vi "validate line configuration.vi"(7 "module":refnum<class "PID Module configuration.lvclass">, 10 "old loop in (optional)":T1={"Loop ID"="", "Tags"={"Setpoint"="", "Process Variable"="", "Output"=""}, "Gains"={"P"=1.0, "I"=0.01, "D"=0.0}, "Range"={"High"=100.0, "Low"=-100.0}}, 11 "new loop in":T1={"Loop ID"="", "Tags"={"Setpoint"="", "Process Variable"="", "Output"=""}, "Gains"={"P"=1.0, "I"=0.01, "D"=0.0}, "Range"={"High"=100.0, "Low"=-100.0}}) -> (1 "valid?":bool, 2 "errors":string, 3 "new loop out":T1={"Loop ID"="", "Tags"={"Setpoint"="", "Process Variable"="", "Output"=""}, "Gains"={"P"=1.0, "I"=0.01, "D"=0.0}, "Range"={"High"=100.0, "Low"=-100.0}})   [LabVIEW 2013, in "PID Module editor node.lvclass"]
uses:
  PID Module editor node.lvclass
  PID array element.ctl
  module/configuration/PID Module configuration.lvclass
  module/configuration/PID Loop/PID Loop.lvclass
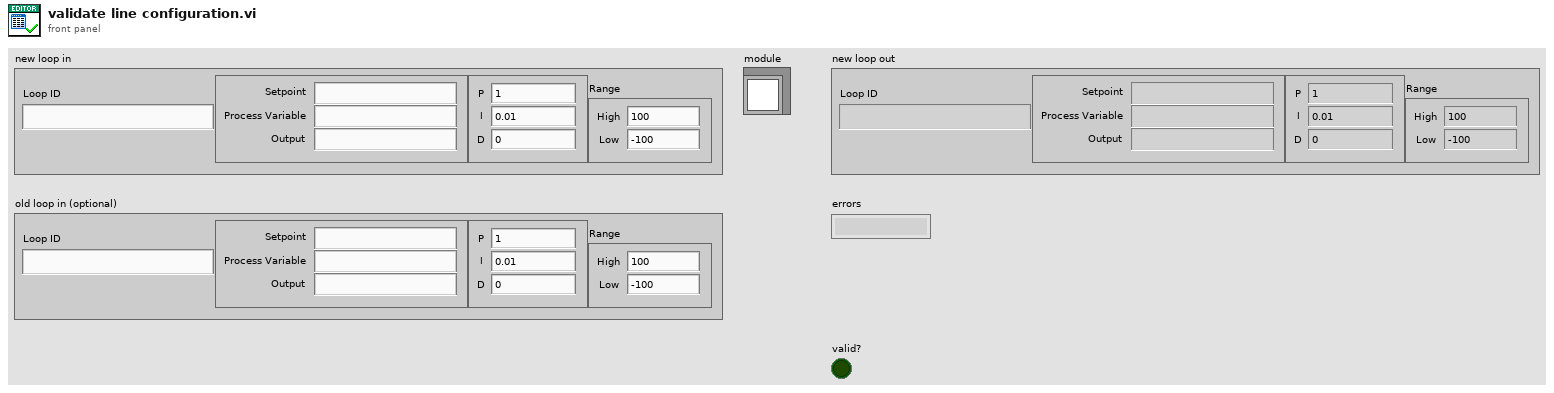
[diagram p1: front panel]
types:
  T1 = typedef "PID Module configuration.lvclass/PID array element.ctl" = cluster{"Loop ID":string, "Tags":cluster{"Setpoint":string, "Process Variable":string, "Output":string}, "Gains":cluster{"P":dbl, "I":dbl, "D":dbl}, "Range":cluster{"High":dbl, "Low":dbl}}
  T2 = typedef "PID Loop.lvclass/PID Parameters.ctl" = cluster{"Setpoint Tag":string, "Process Variable Tag":string, "Output Tag":string}
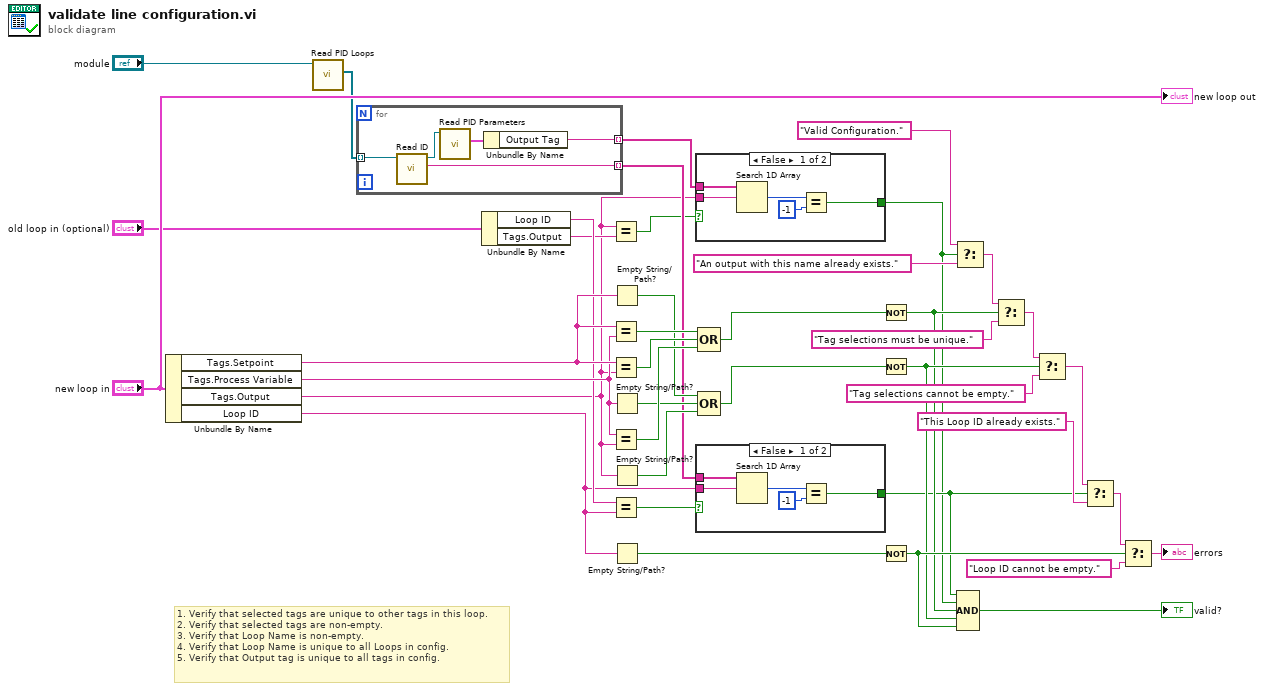
[diagram p0: block diagram]
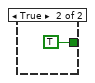
[diagram p2: hidden frame]
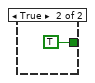
[diagram p3: hidden frame]
diagram:
  # "1. Verify that selected tags are unique to other tags in this loop.\n2. Verify that selected tags are non-empty.\n3. Verify that Loop Name is non-empty.\n4. Verify that Loop Name is unique to all Loops in config.\n5. Verify that Output tag is unique to all tags in config."
  n1 = Unbundle By Name("new loop in") -> ("Tags.Setpoint"=w36:string, "Tags.Process Variable"=w35:string, "Tags.Output"=w4:string, "Loop ID"=w7:string)
  n2 = call-dynamic "Read PID Loops.vi"("Tagbus PID Module configuration in"="module") -> ("PID Loops"=w1:refnum<class "PID Loop.lvclass">[])  [unwired: 8 in, 2 out]
  n3 = for {
    tunnel: w1 -> [w44] mode=indexing
    tunnel: [w43] -> w13 mode=indexing
    tunnel: [w45] -> w11 mode=indexing
    n4 = call-dynamic "Read ID.vi"("PID Loop in"=w44) -> ("ID"=w43:string, "PID Loop out"=w42:refnum<class "PID Loop.lvclass">)  [unwired: 8 in, 1 out]
    n5 = call-dynamic "Read PID Parameters.vi"("PID Loop in"=w42) -> ("PID Parameters"=w41:T2)  [unwired: 8 in, 2 out]
    n6 = Unbundle By Name(w41) -> ("Output Tag"=w45:string)
  }
  n7 = Unbundle By Name("old loop in (optional)") -> ("Loop ID"=w8:string, "Tags.Output"=w5:string)
  n8 = Equal?(x=w4, y=w5) -> (x = y?=w3:bool)
  n9 = Equal?(x=w36, y=w35) -> (x = y?=w39:bool)
  n10 = Equal?(x=w36, y=w4) -> (x = y?=w38:bool)
  n11 = Equal?(x=w35, y=w4) -> (x = y?=w37:bool)
  n12 = Equal?(x=w8, y=w7) -> (x = y?=w6:bool)
  n13 = Empty String/Path?(string/path=w36) -> (empty?=w31:bool)
  n14 = Empty String/Path?(string/path=w35) -> (empty?=w32:bool)
  n15 = Empty String/Path?(string/path=w4) -> (empty?=w33:bool)
  n16 = Empty String/Path?(string/path=w7) -> (empty?=w29:bool)
  n17 = case shown="False" w3 {
    tunnel: w11 -> [w50 _]
    tunnel: w4 -> [w49 _]
    tunnel: [w46 TRUE] -> w10
    frame False {
      n18 = Search 1D Array(1D array=w50, element=w49) -> (index of element=w48:i32)  [unwired: 1 in]
      n19 = Equal?(x=w48, y=-1) -> (x = y?=w46:bool)
    }
    frame True {
    }
  }
  n20 = case shown="False" w6 {
    tunnel: w13 -> [w56 _]
    tunnel: w7 -> [w55 _]
    tunnel: [w52 TRUE] -> w12
    frame False {
      n21 = Search 1D Array(1D array=w56, element=w55) -> (index of element=w54:i32)  [unwired: 1 in]
      n22 = Equal?(x=w54, y=-1) -> (x = y?=w52:bool)
    }
    frame True {
    }
  }
  n23 = Compound Arithmetic op=OR(w39, w38, w37) -> (w34:bool)
  n24 = Compound Arithmetic op=OR(w31, w32, w33) -> (w30:bool)
  n25 = Not(x=w34) -> (.not. x?=w15:bool)
  n26 = Not(x=w30) -> (.not. x?=w16:bool)
  n27 = Not(x=w29) -> (.not. x?=w17:bool)
  n28 = Select(t="Valid Configuration.", s=w10, f="An output with this name already exists.") -> (s? t:f=w18:string)
  n29 = Compound Arithmetic op=AND(w12, w10, w15, w16, w17) -> (→"valid?":bool)
  n30 = Select(t=w18, s=w15, f="Tag selections must be unique.") -> (s? t:f=w21:string)
  n31 = Select(t=w21, s=w16, f="Tag selections cannot be empty.") -> (s? t:f=w22:string)
  n32 = Select(t=w22, s=w12, f="This Loop ID already exists.") -> (s? t:f=w26:string)
  n33 = Select(t=w26, s=w17, f="Loop ID cannot be empty.") -> (s? t:f=→"errors":string)
  "new loop out" <- "new loop in"
